vi "Set Re-entrancy for VIs in a Folder.vi"(6 "Exclude Pattern":string="LV2", 8 "error in (no error)":errorcluster, 9 "Reentrancy Type":T1(ring), 10 "Is Reentrant?":bool=TRUE, 11 "VI Folder":path) -> (0 "error out":errorcluster, 2 "VIs with Errors":path[](array[path]), 3 "VI List":path[](array[path]))   [LabVIEW 2016, in "SLL Scripting.lvlib"]
doc: "This VI can be used to set the re-entrancy setting for all VIs in a folder, with an option to exclude some VIs based on match pattern for the VI name (like LV2s)"
uses:
  SLL Scripting.lvlib
  <vilib>/regexp/Match Regular Expression.xnode
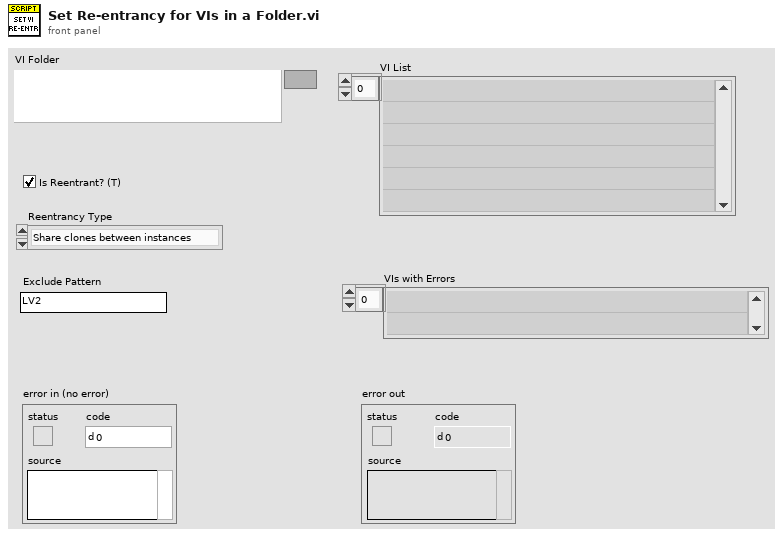
[diagram p1: front panel]
types:
  T1 = enum16{"Share clones between instances", "Preallocate clone for each instance"}
  T2 = enum32{"invalid VI type", "Standard VI", "Control VI", "Global VI", "Polymorphic VI", "Configuration VI", "SubSystem", "Facade VI", "Method VI", "Statechart Diagram VI"}
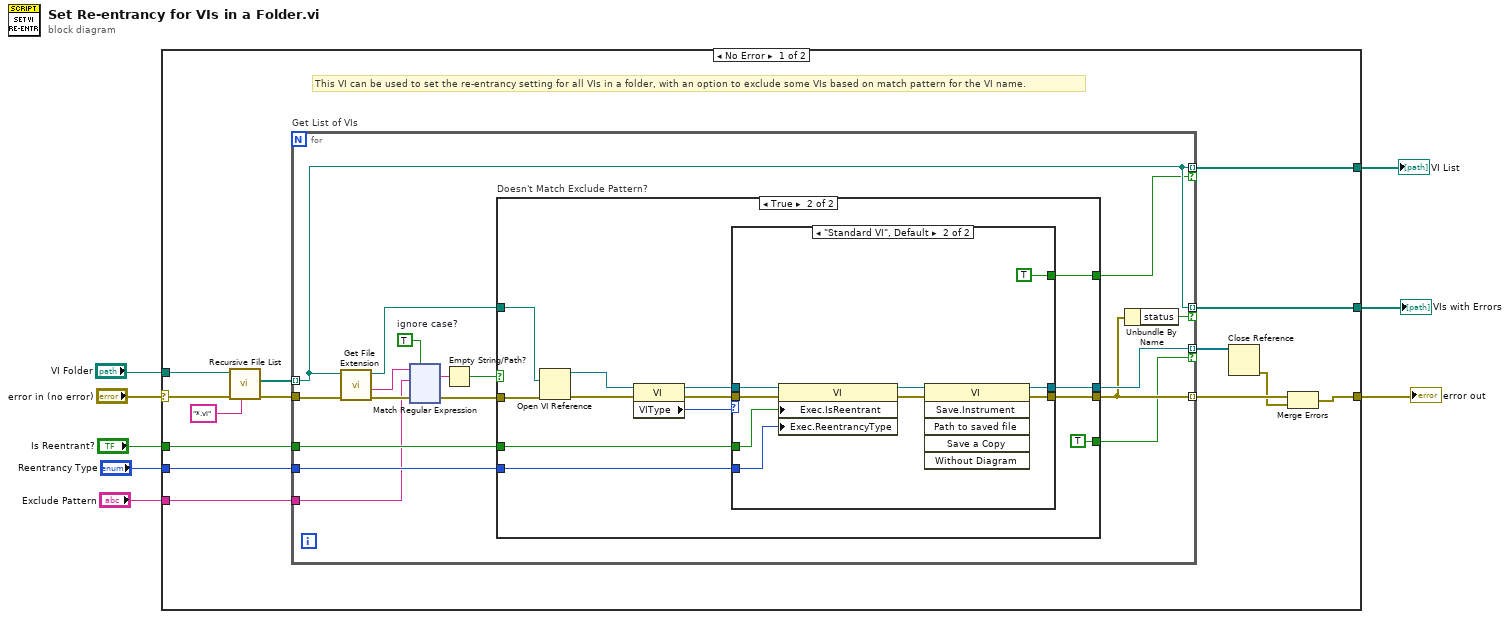
[diagram p0: block diagram]
diagram:
  n1 = case shown="No Error" "error in (no error)" {
    selector: "error in (no error)" -> [w17 w179]
    tunnel: "VI Folder" -> [w21 _]
    tunnel: [w18 _] -> w7
    tunnel: [w13 w179] -> w5
    tunnel: "Reentrancy Type" -> [w12 _]
    tunnel: "Is Reentrant?" -> [w11 _]
    tunnel: [w10 _] -> w2
    tunnel: "Exclude Pattern" -> [w9 _]
    frame No Error {
      # "This VI can be used to set the re-entrancy setting for all VIs in a folder, with an option to exclude some VIs based on match pattern for the VI name."
      n2 = call <vilib>:"Recursive File List.vi"("pattern"="*.vi", "error in (no error)"=w17, "Folder Path"=w21) -> ("error out"=w16:errorcluster, "All Files in Dir"=w19:path[])  [unwired: 4 in, 3 out]
      n3 = for "Get List of VIs" {
        tunnel: [w39] -> w22 mode=indexing if=w23
        tunnel: w19 -> [w33] mode=indexing
        tunnel: [w33] -> w18 mode=indexing if=w24
        tunnel: w16 -> [w34]
        tunnel: [w36] -> w15 mode=indexing
        tunnel: w12 -> [w38]
        tunnel: w11 -> [w37]
        tunnel: [w33] -> w10 mode=indexing if=w35
        tunnel: w9 -> [w27]
        w29 = TRUE  # ignore case?
        n4 = call <vilib>:"Get File Extension.vi"("error in (no error)"=w34, "file"=w33) -> ("error out"=w31:errorcluster, "filename without extension"=w28:string, "dup file"=w32:path)  [unwired: 5 in, 2 out]
        n5 = xnode "Match Regular Expression"("input string"=w28, "regular expression"=w27, "error in"=w31, "ignore case? (F)"=w29) -> ("whole match"=w26:string, "error out"=w30:errorcluster)  [unwired: 2 in, 3 out]
        n6 = Empty String/Path?(string/path=w26) -> (empty?=w25:bool)
        n7 = case "Doesn't Match Exclude Pattern?" shown="True" w25 {
          tunnel: [_ w167] -> w39
          tunnel: w38 -> [_ w166]
          tunnel: w37 -> [_ w165]
          tunnel: [w154 w164] -> w36
          tunnel: w32 -> [_ w163]
          tunnel: w30 -> [w154 w162]
          tunnel: [_ w156] -> w24
          tunnel: [_ TRUE] -> w23
          frame False {
          }
          frame True {
            n8 = Open VI Reference(vi path=w163, error in (no error)=w162) -> (vi reference=w160:refnum<vi>, error out=w161:errorcluster)  [unwired: 4 in]
            n9 = property class="VI"(reference=w160, error in=w161) -> (reference out=w159:refnum<vi>, error out=w158:errorcluster, "VIType"=w157:T2)
            n10 = case shown="\"Standard VI\", Default" w157 {
              tunnel: [w168 w176] -> w167
              tunnel: w166 -> [_ w175]
              tunnel: w165 -> [_ w174]
              tunnel: [w169 w173] -> w164
              tunnel: w159 -> [w168 w172]
              tunnel: w158 -> [w169 w171]
              tunnel: [_ TRUE] -> w156
              frame "Polymorphic VI" {
                # "Note: Polymorphic VIs will result in error when setting the re-entrancy setting"
                # "Ignoring for Polymorphic VIs"
              }
              frame "Standard VI", Default {
                n11 = property class="VI"(reference=w172, error in=w171, "Exec.IsReentrant"=w174, "Exec.ReentrancyType"=w175) -> (reference out=w177:refnum<vi>, error out=w178:errorcluster)
                n12 = invoke class="VI" method="Save.Instrument"(reference=w177, error in=w178) -> (reference out=w176:refnum<vi>, error out=w173:errorcluster)  [unwired: 4 in, 4 out]
              }
            }
          }
        }
        n13 = Unbundle By Name(w36) -> ("status"=w35:bool)
      }
      n14 = Close Reference(reference=w22) -> (error out=w14:errorcluster)  [unwired: 1 in]
      n15 = Merge Errors(w15, w14) -> (w13:errorcluster)
    }
    frame Error {
    }
  }
  "error out" <- w5
  "VI List" <- w7
  "VIs with Errors" <- w2
